vi "Elevator Controller.vi"(8 "error in":errorcluster) -> ()   [LabVIEW 2018]
doc: "This VI executes continuously carrying out the current operation and responding to updates or new operations. It will often contain the timing or control code that is difficult to place directly in TeleOp. This VI generally opens all sensors and motors and isolates the rest of the robot code from knowing how the operations are carried out."
uses:
  <vilib>/Rock Robotics/WPI/Framework/Completion Status.ctl
  Elevator Setpoints.ctl
  Elevator Operations.ctl
  Private/Typedef/Elevator Settings.ctl
  <vilib>/Rock Robotics/WPI/ThirdParty/REV Robotics/SPARK MAX/Typedef/Spark MAX Smart Motion Parameters.ctl
  Private/Typedef/Controller Data.ctl
  <vilib>/Rock Robotics/WPI/MotorControl/WPI_MotorControlDeviceRef.ctl
  <vilib>/Rock Robotics/WPI/MotorControl/WPI_MotorControlType.ctl
  <vilib>/Rock Robotics/SystemInterfaces/DIO/FPGA_DIOPWMChannel.ctl
  <vilib>/Rock Robotics/WPI/PWM/WPI_PWMDeadband.ctl
  <vilib>/Rock Robotics/SystemInterfaces/DIO/FPGA_DIOChannel.ctl
  Elevator Telemetry.ctl
  <vilib>/Rock Robotics/Network Tables/NT Write Number.vi
  Elevator Published Globals.vi
panel:
  out "Is Moving?":bool=TRUE
  out "PID Chart":T1(graph)={"Sensor Velocity"=-0.0, "Setpoint"=14.047639846801758, "Sensor Position"=10.690532684326172, "Applied Output"=-0.0}
  in  "Settings":T2={"min speed"=0.0, "Position Max"=69.0, "gravity"=1.25, "PID Constants"={"P Gain"=5e-05, "I Gain"=0.0, "D Gain"=1e-05, "F Gain"=0.00015, "I Zone"=0.0, "Min Output"=-1.0, "Max Output"=1.0}, "SM Params"={"Max Velocity"=6200.0, "Max Acceleration"=12000.0, "Minimum Velocity Output"=0.0, "Allowed Closed Loop Error"=0.01}} {"gravity" format="%#_13g"; "Position Max" format="%#_13g"; "min speed" format="%#_13g"}
  out "Switches":T4
  in  "Interactive Values":T5={"Operation"=enum."Go to Position", "Setpoint"=0.0, "Duration"=0.0}
  out "Current\nCmd":string="Started at  09:23:59.692\nDefault: Reserve,  S 0.0, D 0.000000"
  in  "Buttons":cluster{"Execute Cmd":bool, "Abort Cmd":bool}
  out "Command Timing":cluster{"Start Time (ms)":u32, "Iterations":i32}={"Start Time (ms)"=2681160, "Iterations"=0}
  out "Status":T7
  # "Interactive Command: You may fill in the settings for a command\nand schedule it with the Execute button. You can observe and abort\nany command while fine tuning the code for the controller."
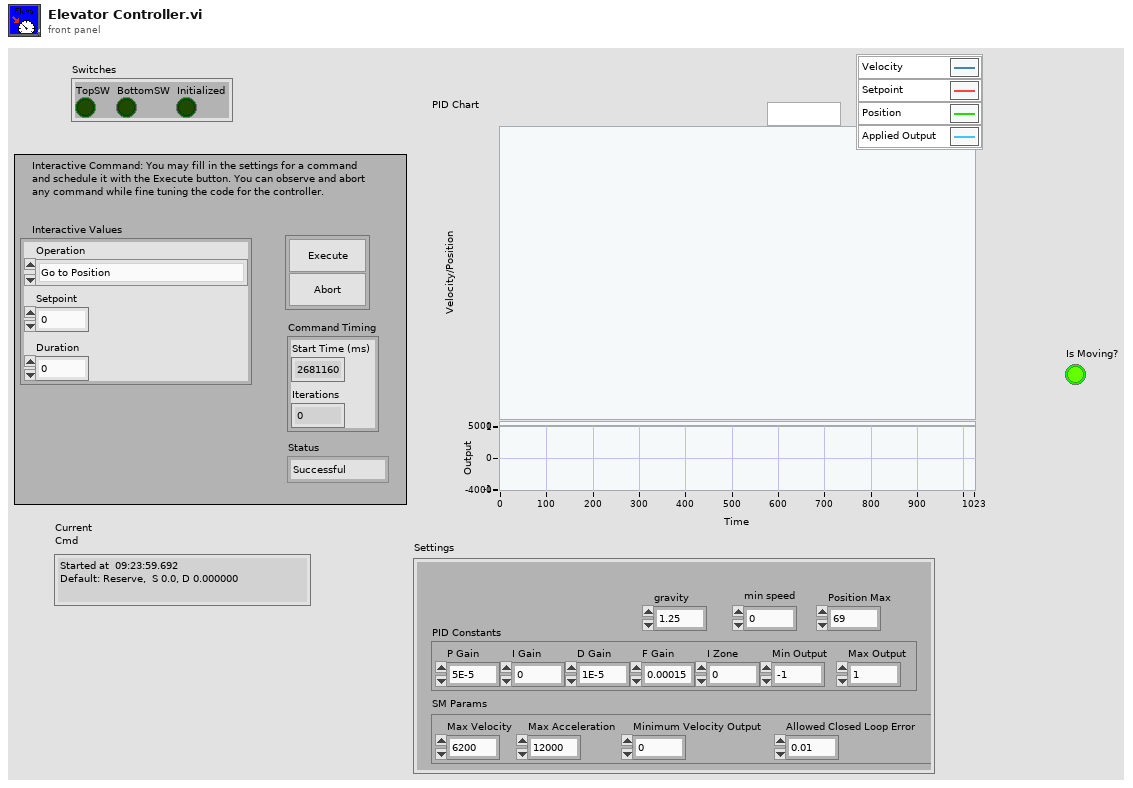
[diagram p1: front panel]
types:
  T1 = cluster{"Sensor Velocity":dbl, "Setpoint":dbl, "Sensor Position":dbl, "Applied Output":dbl}
  T2 = typedef "Elevator Settings.ctl" = cluster{"min speed":dbl, "Position Max":dbl, "gravity":dbl, "PID Constants":cluster{"P Gain":dbl, "I Gain":dbl, "D Gain":dbl, "F Gain":dbl, "I Zone":dbl, "Min Output":dbl, "Max Output":dbl}, "SM Params":T3}
  T3 = typedef "Spark MAX Smart Motion Parameters.ctl" = cluster{"Max Velocity":dbl, "Max Acceleration":dbl, "Minimum Velocity Output":dbl, "Allowed Closed Loop Error":dbl}
  T4 = cluster{"TopSW":bool, "BottomSW":bool, "Initialized":bool}
  T5 = typedef "Elevator Setpoints.ctl" = cluster{"Operation":T6, "Setpoint":dbl, "Duration":dbl}
  T6 = typedef "Elevator Operations.ctl" = enum16{"Reserve", "Read Current", "Immediate", "Stop", "Switch", "Scale", "Home", "Go to Position", "Set Max Height"}
  T7 = typedef "Completion Status.ctl" = enum16{"Successful", "Aborted", "Incomplete"}
  T8 = typedef "Controller Data.ctl" = cluster{"Setpoint":dbl, "Output":dbl, "DriveMotor1":T9, "Is Done Moving?":bool}
  T9 = typedef "WPI_MotorControlDeviceRef.ctl" = cluster{"DeviceStatus":errorcluster, "Type":T10, "PWM":cluster{"PWM Channel":T11, "DeadBand":T12}, "CAN":cluster{"Device Number":u8, "SetOutput VI Ref":variant, "GetOutput VI Ref":variant, "Enable VI Ref":variant, "Disable VI Ref":variant, "Data":variant}, "Invert":bool, "DIO PWM":cluster{"PWM \"Enable\" Channel":T11, "DIOChannel":T13, "PWM Rate":dbl}}
  T10 = typedef "WPI_MotorControlType.ctl" = enum16{"PWM", "CAN", "DIO PWM"}
  T11 = typedef "FPGA_DIOPWMChannel.ctl" = enum8{"PWM 0", "PWM 1", "PWM 2", "PWM 3", "PWM 4", "PWM 5", "PWM 6", "PWM 7", "PWM 8", "PWM 9", "PWM MXP 0", "PWM MXP 1", "PWM MXP 2", "PWM MXP 3", "PWM MXP 4", "PWM MXP 5", "PWM MXP 6", "PWM MXP 7", "PWM MXP 8", "PWM MXP 9", "Invalid"}
  T12 = typedef "WPI_PWMDeadband.ctl" = cluster{"Name":string, "maxPositivePwm":i32, "minPositivePwm":i32, "centerPwm":i32, "maxNegativePwm":i32, "minNegativePwm":i32, "angularRange":u16}
  T13 = typedef "FPGA_DIOChannel.ctl" = enum8{"DIO 0", "DIO 1", "DIO 2", "DIO 3", "DIO 4", "DIO 5", "DIO 6", "DIO 7", "DIO 8", "DIO 9", "DIO MXP 0", "DIO MXP 1", "DIO MXP 2", "DIO MXP 3", "DIO MXP 4", "DIO MXP 5", "DIO MXP 6", "DIO MXP 7", "DIO MXP 8", "DIO MXP 9", "DIO MXP 10", "DIO MXP 11", "DIO MXP 12", "DIO MXP 13", "DIO MXP 14", "DIO MXP 15", "SPI Port CS1", "SPI Port CS2", "SPI Port CS3", "SPI Port MISO", "SPI Port MOSI", "Invalid"}
  T14 = typedef "Command Status Info.ctl" = cluster{"Name":string, "Status":T7, "notifier out":T15}
  T15 = typedef "Completion Notifier.ctl" = refnum<notifier>
  T16 = cluster{"Current Command":T5, "Command Timing":cluster{"Start Time (ms)":u32, "Iterations":i32}, "Command Arguments":cluster{"Command Info":T14, "Description":string, "Default Command":T5, "queue out":refnum<queue>, "Subsystem Name":string}}
  T17 = typedef "Elevator Telemetry.ctl" = cluster{"Is Moving?":bool, "Setpoint":dbl, "Velocity":dbl, "Position":dbl, "Top Limit":bool, "Bottom Limit":bool, "Applied Output":dbl}
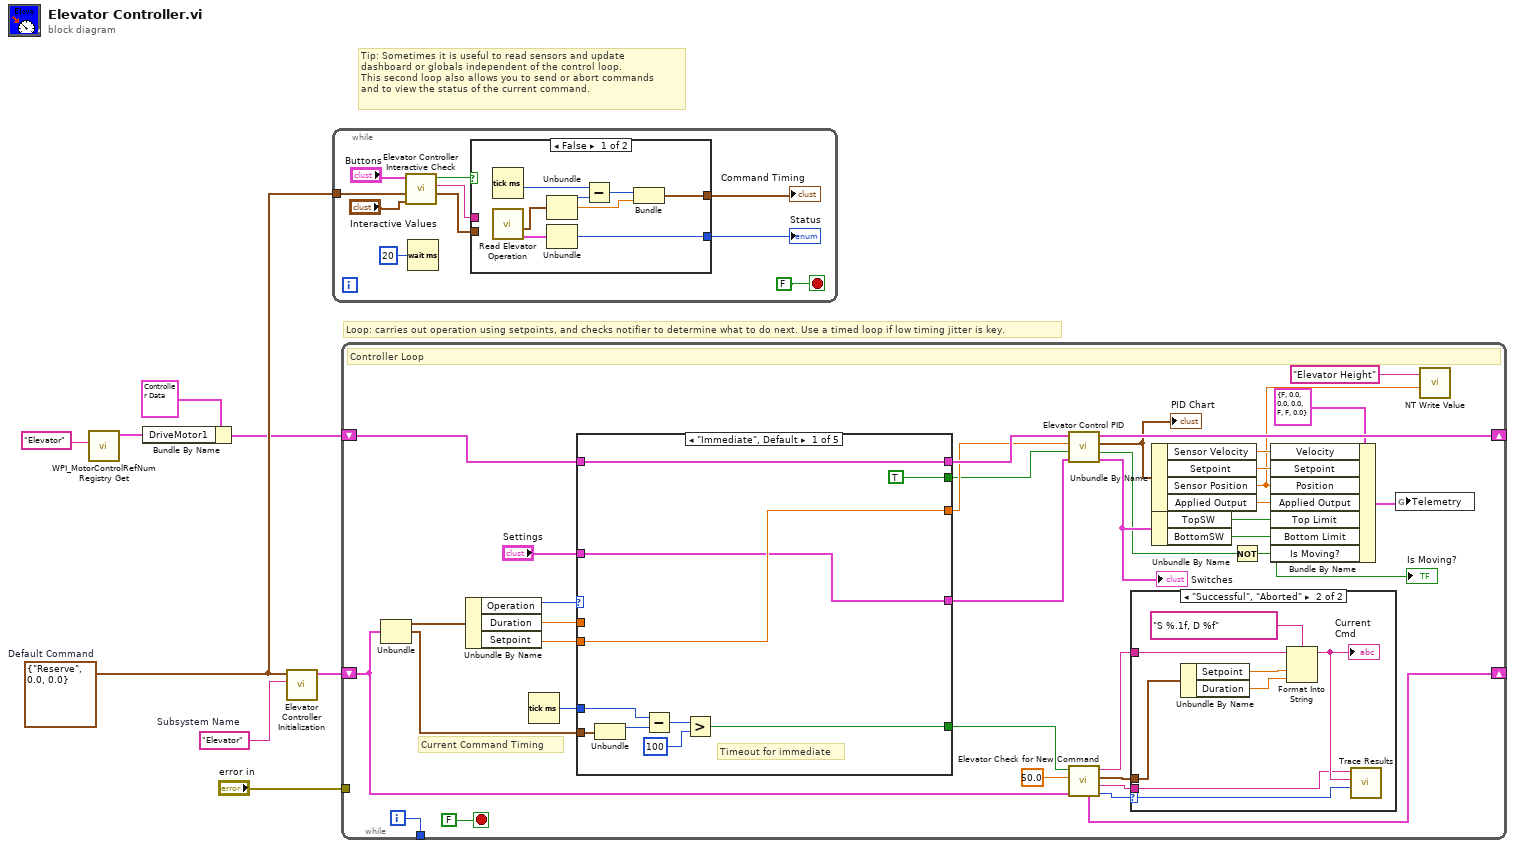
[diagram p0: block diagram]
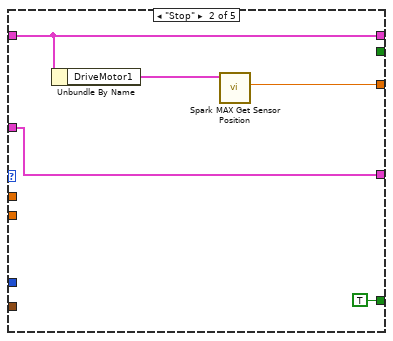
[diagram p2: hidden frame]
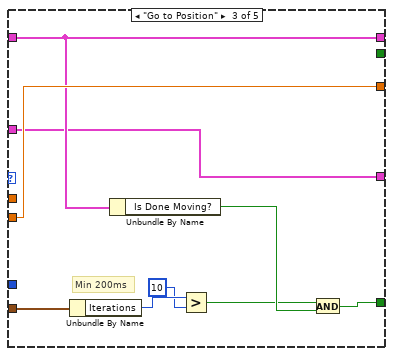
[diagram p3: hidden frame]
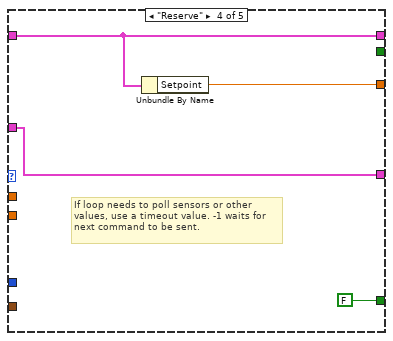
[diagram p4: hidden frame]
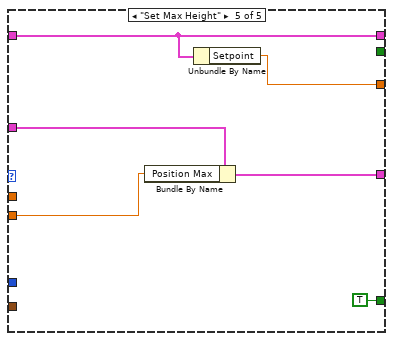
[diagram p5: hidden frame]
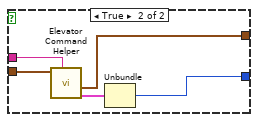
[diagram p7: hidden frame]
diagram:
  w6 = T5 {"Operation"=enum."Reserve", "Setpoint"=0.0, "Duration"=0.0}  # Default Command
  w7 = "Elevator"  # Subsystem Name
  # "Tip: Sometimes it is useful to read sensors and update\ndashboard or globals independent of the control loop.\nThis second loop also allows you to send or abort commands\nand to view the status of the current command."
  # "Loop: carries out operation using setpoints, and checks notifier to determine what to do next. Use a timed loop if low timing jitter is key."
  n1 = call <vilib>:"WPI_MotorControlRefNum Registry Get.vi"("refnum name"="Elevator") -> ("MotorControlDevRef"=w3:T9)  [unwired: 9 in, 1 out]
  n2 = Bundle By Name(cluster=T8 {"Setpoint"=0.0, "Output"=0.0, "DriveMotor1"={"DeviceStatus"={"status"=FALSE, "code"=0, "source"=""}, "Type"=enum."PWM", "PWM"={"PWM Channel"=enum."Invalid", "DeadBand"={"Name"="", "maxPositivePwm"=0, "minPositivePwm"=0, "centerPwm"=0, "maxNegativePwm"=0, "minNegativePwm"=0, "angularRange"=0}}, "CAN"={"Device Number"=0, "SetOutput VI Ref"=variant(enum8{"Percent VBus", "Current", "Speed", "Position", "Voltage"} enum."Percent VBus"), "GetOutput VI Ref"=variant(refnum<k1> refnum), "Enable VI Ref"=variant(dbl 12.0), "Disable VI Ref"=variant(enum8{"Percent VBus", "Speed", "Position", "Slave", "Unchanged / Invalid"} enum."Percent VBus"), "Data"=variant(enum16{"Controller 1"} enum."Controller 1")}, "Invert"=FALSE, "DIO PWM"={"PWM \"Enable\" Channel"=enum."Invalid", "DIOChannel"=enum."Invalid", "PWM Rate"=0.0}}, "Is Done Moving?"=FALSE}, "DriveMotor1"=w3) -> (w2:T8)
  n3 = call "Elevator Controller Initialization.vi"("Subsystem Name"=w7, "Default Command"=w6) -> ("Current Command"=w5:T16)  [unwired: 9 in]
  n4 = while {
    tunnel: w6 -> [w15]
    stop <- FALSE stop-if-true
    n5 = call "Elevator Controller Interactive Check.vi"("Interactive Command in"="Interactive Values", "Default Command"=w15, "Buttons"="Buttons") -> ("Interactive Command out"=w12:T5, "Trace String"=w13:string, "Schedule"=w14:bool)  [unwired: 6 in]
    n6 = Wait (ms)(milliseconds to wait=u32 20) -> ()  [unwired: 1 out]
    n7 = case shown="False" w14 {
      tunnel: [w26 w31] -> w11
      tunnel: w12 -> [_ w29]
      tunnel: [w22 w27] -> w10
      tunnel: w13 -> [_ w30]
      frame False {
        n8 = Tick Count (ms)() -> (millisecond timer value=w21:u32)
        n9 = call "Read Elevator Operation.vi"() -> ("Command Info"=w19:T14, "SubSystem Data"=w20:T5)  [unwired: 9 in, 1 out]
        n10 = Unbundle(w20) -> ("Operation"=w25:T6, "Setpoint"=w23:dbl)  [unwired: 1 out]
        n11 = Unbundle(w19) -> ("Status"=w26:T7)  [unwired: 2 out]
        n12 = Subtract(x=w21, y=w25) -> (x-y=w24:u32)
        n13 = Bundle(w24, "Setpoint"=w23) -> (w22:cluster{u32, "Setpoint":dbl})  [unwired: 1 in]
      }
      frame True {
        n14 = call "Elevator Command Helper.vi"("Description"=w30, "SubSystem Data"=w29) -> ("Command Info Out"=w28:T14, "Command Timing"=w27:cluster{"Start Time (ms)":u32, "Iterations":i32})  [unwired: 7 in, 1 out]
        n15 = Unbundle(w28) -> ("Status"=w31:T7)  [unwired: 2 out]
      }
    }
    "Status" <- w11
    "Command Timing" <- w10
  }
  n16 = while {
    shift-right: [w59] -> _
    shift-left: w5 -> [w53]
    tunnel: [w66] -> _
    tunnel: "error in" -> [_]
    shift-right: [w50] -> _
    shift-left: w2 -> [w52]
    i -> [w66]
    stop <- FALSE stop-if-true
    # "Current Command Timing"
    # "Controller Loop"
    n17 = Unbundle(w53) -> ("Current Command"=w65:T5, "Command Timing"=w61:cluster{"Start Time (ms)":u32, "Iterations":i32})  [unwired: 1 out]
    n18 = Unbundle By Name(w65) -> ("Operation"=w64:T6, "Duration"=w63:dbl, "Setpoint"=w60:dbl)
    n19 = Tick Count (ms)() -> (millisecond timer value=w62:u32)
    n20 = case shown="\"Immediate\", Default" w64 {
      tunnel: [w72 TRUE ("ignore previous (F)") w85 FALSE ("ignore previous (F)") TRUE ("ignore previous (F)")] -> w58
      tunnel: w61 -> [w74 _ w88 _ _]
      tunnel: w63 -> [_ _ _ _ _]
      tunnel: w62 -> [w73 _ _ _ _]
      tunnel: w60 -> [w69 _ w91 _ w98]
      tunnel: w52 -> [w71 w82 w90 w94 w97]
      tunnel: [w71 w82 w90 w94 w97] -> w51
      tunnel: [w69 w79 w91 w93 w96] -> w49
      tunnel: [TRUE _ _ _ _] -> w48
      tunnel: "Settings" -> [w68 w78 w83 w92 w100]
      tunnel: [w68 w78 w83 w92 w99] -> w32
      frame "Immediate", Default {
        # "Timeout for immediate"
        n21 = Unbundle(w74) -> ("Start Time (ms)"=w77:u32)  [unwired: 1 out]
        n22 = Subtract(x=w73, y=w77) -> (x-y=w76:u32)
        n23 = Greater?(x=w76, y=u8 100 ("Left Motor")) -> (0:w72:bool)
      }
      frame "Stop" {
        n24 = Unbundle By Name(w82) -> ("DriveMotor1"=w80:T9)
        n25 = call <vilib>:"Spark MAX Get Sensor Position.vi"("MotorControlDevRef in"=w80) -> ("Sensor Position"=w79:dbl)  [unwired: 7 in, 3 out]
      }
      frame "Go to Position" {
        # "Min 200ms"
        n26 = Unbundle By Name(w88) -> ("Iterations"=w87:i32)
        n27 = Unbundle By Name(w90) -> ("Is Done Moving?"=w89:bool)
        n28 = Greater?(x=w87, y=10 ("x")) -> (0:w84:bool)
        n29 = And(x=w84, y=w89) -> (x .and. y?=w85:bool)
      }
      frame "Reserve" {
        # "If loop needs to poll sensors or other\nvalues, use a timeout value. -1 waits for\nnext command to be sent."
        n30 = Unbundle By Name(w94) -> ("Setpoint"=w93:dbl)
      }
      frame "Set Max Height" {
        n31 = Bundle By Name(cluster=w100, "Position Max"=w98) -> (w99:T2)
        n32 = Unbundle By Name(w97) -> ("Setpoint"=w96:dbl)
      }
    }
    n33 = call "Elevator Control PID.vi"("Settings"=w32, "Manual"=w48, "Setpoint"=w49, "Controller In"=w51) -> ("Switches"=w43:T4, "Path is Done?"=w37:bool, "PID Chart"=w44:T1, "Controller out"=w50:T8)  [unwired: 4 in]
    "Switches" <- w43
    "PID Chart" <- w44
    n34 = call "Elevator Check for New Command.vi"("Current Command"=w53, "Wait time (ms)"=50.0, "Finished?"=w58) -> ("Completion"=w54:T7, "Subsystem Name"=w55:string, "Current Command"=w56:T5, "Initial Trace String"=w57:string, "NextCommand"=w59:T16)  [unwired: 4 in]
    n35 = case shown="\"Successful\", \"Aborted\"" w54 {
      selector: w54 -> [_ w102]
      tunnel: w57 -> [_ w106]
      tunnel: w56 -> [_ w107]
      tunnel: w55 -> [_ w103]
      frame "Incomplete", Default {
        # "Continuing current command"
      }
      frame "Successful", "Aborted" {
        # "Report and setup for next command"
        n36 = Unbundle By Name(w107) -> ("Setpoint"=w109:dbl, "Duration"=w104:dbl)
        n37 = Format Into String(format string="S %.1f, D %f", initial string=w106, w109, w104) -> (resulting string=w105:string)  [unwired: 1 in, 1 out]
        "Current\nCmd" <- w105
        n38 = call <vilib>:"Trace Results.vi"("Status of previous command"=w102, "Description"=w105, "Subsystem"=w103) -> ()  [unwired: 9 in]
      }
    }
    n39 = Unbundle By Name(w44) -> ("Sensor Velocity"=w38:dbl, "Setpoint"=w39:dbl, "Sensor Position"=w35:dbl, "Applied Output"=w40:dbl)
    n40 = Unbundle By Name(w43) -> ("TopSW"=w42:bool, "BottomSW"=w41:bool)
    n41 = Not(x=w37) -> (.not. x?=w36:bool)
    "Is Moving?" <- w36
    n42 = Bundle By Name(cluster=T17 {"Is Moving?"=FALSE, "Setpoint"=0.0, "Velocity"=0.0, "Position"=0.0, "Top Limit"=FALSE, "Bottom Limit"=FALSE, "Applied Output"=0.0} ("Telemetry"), "Velocity"=w38, "Setpoint"=w39, "Position"=w35, "Applied Output"=w40, "Top Limit"=w42, "Bottom Limit"=w41, "Is Moving?"=w36) -> (w45:T17)
    n43 = global write "Elevator Published Globals.vi" "Telemetry"(w45) -> ()
    n44 = call-poly <vilib>:"NT Write Value.vi"("Numeric"=w35, "Name"="Elevator Height") -> ()  [unwired: 9 in, 1 out]
  }
